vi "1L20_conv_degre_Kelvin.vi"(1 "Deg C":dbl format="%.2f") -> (0 "Deg K":dbl format="%.2f")   [LabVIEW 2010, in "lv_01.lvlib"]
doc: "Conversion de degré Celsius en Kelvin."
uses:
  lv_01.lvlib
panel:
  # "This VI converts a Celsius temperature to Kelvin."
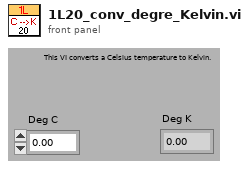
[diagram p1: front panel]
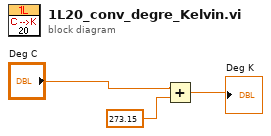
[diagram p0: block diagram]
diagram:
  n1 = Add(x="Deg C", y=273.15) -> (x+y=→"Deg K":dbl)
